vi "Fdx Create Virtual Link (VL).vi"   [LabVIEW 2020, in "AIM664LV.lvlib"]
uses:
  AIM664LV.lvlib
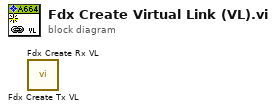
[diagram p0: block diagram]
diagram:
  n1 = call "Fdx Create Tx VL.vi"() -> ()  [unwired: 9 in, 3 out]
  n2 = call "Fdx Create Rx VL.vi"() -> ()  [unwired: 9 in, 3 out]
